vi "Stop Core.vi"(10 "final error code":i32, 11 "Shaker Controller in":refnum<class "Shaker Controller.lvclass">) -> (3 "Shaker Controller out":refnum<class "Shaker Controller.lvclass">)   [LabVIEW 2020, in "Shaker Controller.lvlib" / "Shaker Controller.lvclass"]
doc: "(<B>Filename</B>: Actor Framework.lvlib:Actor.lvclass:Stop Core.vi)\n\nDefines what the actor does before it stops. Use the <B>final error code</B> input to determine whether the actor shut down in response to an error.\n\nBy default, this method passes the Stop message along to all auto-stop nested actors. A descendant class may override this method to define additional behavior, such as shutting down any processes the actor initiated in its override of the Actor Core method."
uses:
  Shaker Controller.lvclass
  Shaker Controller.lvclass/Shaker Controller.ctl
  <vilib>/MGI/Monitored Actor/Monitored Actor/Monitored Actor/Monitored Actor.lvclass
  _Abstract Classes/Abstract Shake Monitor/Abstract Shake Monitor.lvclass
  _Abstract Classes/Abstract Shaker/Abstract Shaker.lvclass
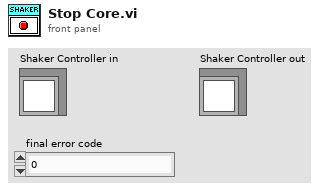
[diagram p1: front panel]
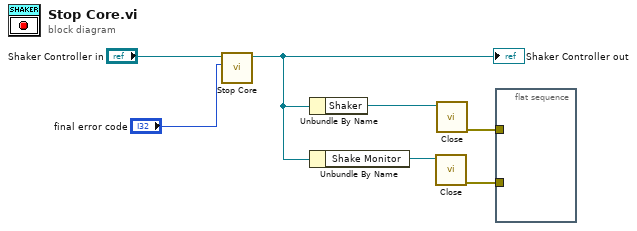
[diagram p0: block diagram]
diagram:
  n1 = call-parent "Stop Core.vi"("final error code"="final error code", "Monitored Actor in"="Shaker Controller in") -> ("Monitored Actor out"=w3:refnum<class "Shaker Controller.lvclass">)  [unwired: 9 in]
  "Shaker Controller out" <- w3
  n2 = Unbundle By Name(w3) -> ("Shaker"=w5:refnum<class "Abstract Shaker.lvclass">)
  n3 = Unbundle By Name(w3) -> ("Shake Monitor"=w2:refnum<class "Abstract Shake Monitor.lvclass">)
  n4 = call-dynamic "Close.vi"("Abstract Shake Monitor in"=w2) -> ("error out"=w1:errorcluster)  [unwired: 9 in, 1 out]
  n5 = call-dynamic "Close.vi"("Abstract Shaker in"=w5) -> ("error out"=w4:errorcluster)  [unwired: 9 in, 1 out]
  n6 = flat-sequence {
    tunnel: w4 -> [_]
    tunnel: w1 -> [_]
    frame #0 {
    }
  }
